vi "Lift_Function.vi"(9 "Input Cluster":T1={"Level 5"=TRUE, "Level 4"=TRUE, "Level 3"=TRUE, "Level 2"=TRUE, "Level 1"=FALSE}, 10 "MotorControlDevRef":T2={"DeviceStatus"={"status"=FALSE, "code"=0, "source"=""}, "Type"=enum."PWM", "PWM"={"Digital Module"=enum."Digital Module 1", "PWM Channel"=enum."Invalid", "DeadBand"={"Name"="", "maxPositivePwm"=0, "minPositivePwm"=0, "centerPwm"=0, "maxNegativePwm"=0, "minNegativePwm"=0, "angularRange"=0}}, "CAN"={"Device Number"=0, "Control Mode"=enum."Percent VBus", "Semaphore"=refnum, "Max Vout"=12.0}, "Invert"=FALSE, "TransformRef"=refnum, "InvTransformRef"=refnum}, 11 "EncoderDevRef":T9={"DevStatus"={"status"=FALSE, "code"=0, "source"=""}, "EncoderIndex"=enum."Invalid", "CounterIndex"=enum."Ctr 1", "DistancePerCount"=2.0, "Decoding Type"=enum."4x"}) -> (3 "Output Cluster":T1)   [LabVIEW 2014]
uses:
  <vilib>/Rock Robotics/SystemInterfaces/Encoder/FPGA_EncoderIdx.ctl
  <vilib>/Rock Robotics/WPI/Encoder/WPI_EncoderType.ctl
  <vilib>/Rock Robotics/SystemInterfaces/Counter/FPGA_CounterCtrSystemIndex.ctl
  <vilib>/Rock Robotics/WPI/Encoder/WPI_EncoderDevRef.ctl
  <vilib>/Rock Robotics/WPI/MotorControl/WPI_MotorControlDeviceRef.ctl
  <vilib>/Rock Robotics/WPI/PWM/WPI_PWMTransform_ConPane.ctl
  <vilib>/Rock Robotics/SystemInterfaces/Typedef/FPGA_TypedefDigitalModule.ctl
  <vilib>/Rock Robotics/SystemInterfaces/DIO/FPGA_DIOPWMChannel.ctl
  <vilib>/Rock Robotics/WPI/PWM/WPI_PWMDeadband.ctl
  <vilib>/Rock Robotics/WPI/CAN/Jaguar/SubVIs/WPI_CANJaguar_ControlMode.ctl
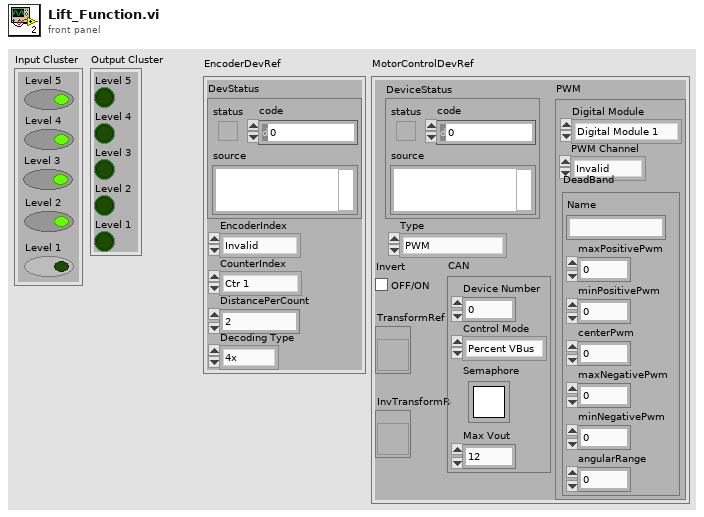
[diagram p1: front panel]
types:
  T1 = cluster{"Level 5":bool, "Level 4":bool, "Level 3":bool, "Level 2":bool, "Level 1":bool}
  T2 = typedef "WPI_MotorControlDeviceRef.ctl" = cluster{"DeviceStatus":errorcluster, "Type":enum16{"PWM", "CAN"}, "PWM":cluster{"Digital Module":T3, "PWM Channel":T4, "DeadBand":T5}, "CAN":cluster{"Device Number":u8, "Control Mode":T6, "Semaphore":T7, "Max Vout":dbl}, "Invert":bool, "TransformRef":T8, "InvTransformRef":T8}
  T3 = typedef "FPGA_TypedefDigitalModule.ctl" = enum16{"Digital Module 1", "Digital Module 2"}
  T4 = typedef "FPGA_DIOPWMChannel.ctl" = enum8{"PWM 1", "PWM 2", "PWM 3", "PWM 4", "PWM 5", "PWM 6", "PWM 7", "PWM 8", "PWM 9", "PWM 10", "Invalid"}
  T5 = typedef "WPI_PWMDeadband.ctl" = cluster{"Name":string, "maxPositivePwm":i32, "minPositivePwm":i32, "centerPwm":i32, "maxNegativePwm":i32, "minNegativePwm":i32, "angularRange":u16}
  T6 = typedef "WPI_CANJaguar_ControlMode.ctl" = enum8{"Percent VBus", "Current", "Speed", "Position", "Voltage"}
  T7 = typedef "Semaphore RefNum" = refnum<k1>
  T8 = typedef "WPI_PWMTransform_ConPane.ctl" = refnum<vi>
  T9 = typedef "WPI_EncoderDevRef.ctl" = cluster{"DevStatus":errorcluster, "EncoderIndex":T10, "CounterIndex":T11, "DistancePerCount":dbl, "Decoding Type":T12}
  T10 = typedef "FPGA_EncoderIdx.ctl" = enum8{"Enc 0", "Enc 1", "Enc 2", "Enc 3", "Invalid"}
  T11 = typedef "FPGA_CounterCtrSystemIndex.ctl" = enum8{"Ctr 0", "Ctr 1", "Ctr 2", "Ctr 3", "Ctr 4", "Ctr 5", "Ctr 6", "Ctr 7", "Invalid"}
  T12 = typedef "WPI_EncoderType.ctl" = enum16{"1x", "2x", "4x"}
  T13 = cluster{"Level":bool, "Level":bool, "Level":bool, "Level":bool, "Level":bool}
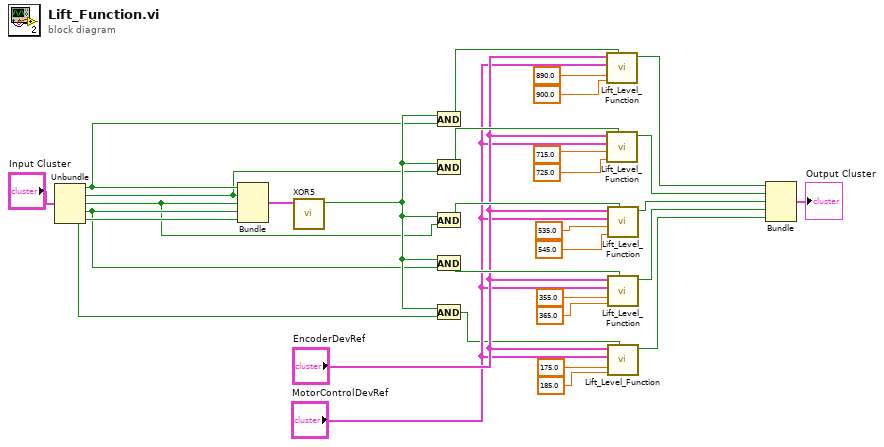
[diagram p0: block diagram]
diagram:
  n1 = Unbundle("Input Cluster") -> ("Level 5"=w5:bool, "Level 4"=w4:bool, "Level 3"=w1:bool, "Level 2"=w2:bool, "Level 1"=w3:bool)
  n2 = Bundle("Level 5"=w5, "Level 4"=w4, "Level 3"=w1, "Level 2"=w2, "Level 1"=w3) -> (w31:T1)  [unwired: 1 in]
  n3 = call "XOR5.vi"("inputs"=w31) -> ("XOR5"=w30:bool)  [unwired: 10 in]
  n4 = And(x=w30, y=w5) -> (x .and. y?=w29:bool)
  n5 = And(x=w30, y=w4) -> (x .and. y?=w28:bool)
  n6 = And(x=w30, y=w1) -> (x .and. y?=w27:bool)
  n7 = And(x=w30, y=w2) -> (x .and. y?=w26:bool)
  n8 = And(x=w30, y=w3) -> (x .and. y?=w15:bool)
  n9 = call "Lift_Level_Function.vi"("Level"=w29, "upper limit"=900.0, "lower Limit"=890.0, "MotorControlDevRef"="MotorControlDevRef", "EncoderDevRef"="EncoderDevRef") -> ("Level"=w12:bool)  [unwired: 6 in]
  n10 = call "Lift_Level_Function.vi"("Level"=w28, "upper limit"=725.0, "lower Limit"=715.0, "MotorControlDevRef"="MotorControlDevRef", "EncoderDevRef"="EncoderDevRef") -> ("Level"=w11:bool)  [unwired: 6 in]
  n11 = call "Lift_Level_Function.vi"("Level"=w27, "upper limit"=545.0, "lower Limit"=535.0, "MotorControlDevRef"="MotorControlDevRef", "EncoderDevRef"="EncoderDevRef") -> ("Level"=w10:bool)  [unwired: 6 in]
  n12 = call "Lift_Level_Function.vi"("Level"=w26, "upper limit"=365.0, "lower Limit"=355.0, "MotorControlDevRef"="MotorControlDevRef", "EncoderDevRef"="EncoderDevRef") -> ("Level"=w9:bool)  [unwired: 6 in]
  n13 = call "Lift_Level_Function.vi"("Level"=w15, "upper limit"=185.0, "lower Limit"=175.0, "MotorControlDevRef"="MotorControlDevRef", "EncoderDevRef"="EncoderDevRef") -> ("Level"=w8:bool)  [unwired: 6 in]
  n14 = Bundle("Level"=w12, "Level"=w11, "Level"=w10, "Level"=w9, "Level"=w8) -> (→"Output Cluster":T13)  [unwired: 1 in]
